vi "Initialize.vi"(8 "error in (no error)":errorcluster, 11 "UDP Thread UI in":refnum<class "UDP Thread User Interface.lvclass">) -> (0 "error out":errorcluster, 3 "UDP Thread UI out":refnum<class "UDP Thread User Interface.lvclass">)   [LabVIEW 2023, in "UDP.lvlib" / "UDP Thread User Interface.lvclass"]
uses:
  UDP Thread User Interface.lvclass
  C:/Users/Public/Documents/National Instruments/NI VeriStand 2023/Custom Devices/Data Sharing Framework/Linux_x64/DSF Core.lvlibp/Classes/User Interface/User Interface.lvclass
  Configuration/Thread/UDP Thread Configuration.lvclass
  C:/Users/Public/Documents/National Instruments/NI VeriStand 2023/Custom Devices/Data Sharing Framework/Linux_x64/DSF Core.lvlibp/Classes/Configuration/Configuration.lvclass
  Users/Public/Documents/National Instruments/NI VeriStand 2023/Custom Devices/Data Sharing Framework/Linux_x64/DSF Core.lvlibp/Classes/User Interface/User Interface.lvclass
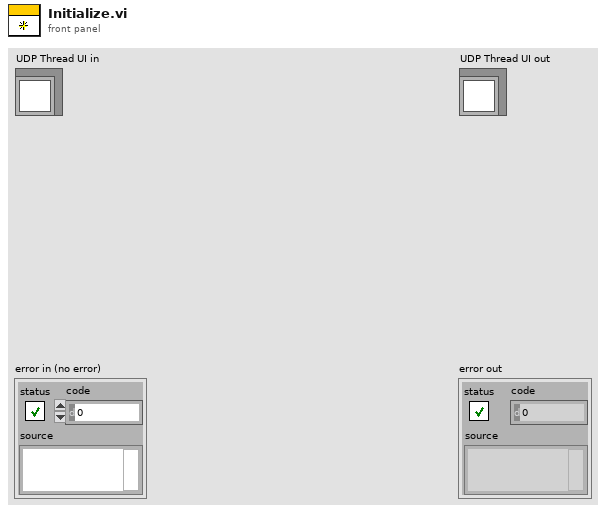
[diagram p1: front panel]
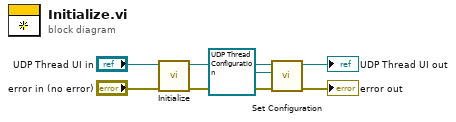
[diagram p0: block diagram]
diagram:
  n1 = call-parent "Initialize.vi"("error in (no error)"="error in (no error)", "User Interface in"="UDP Thread UI in") -> ("error out"=w4:errorcluster, "User Interface out"=w5:refnum<class "UDP Thread User Interface.lvclass">)  [unwired: 8 in]
  n2 = call "Set Configuration.vi"("error in (no error)"=w4, "configuration"=refnum<class "UDP Thread Configuration.lvclass"> refnum ("DSF Core.lvlib:DSF UDP Thread Configuration"), "User Interface in"=w5) -> ("error out"=→"error out":errorcluster, "User Interface out"=→"UDP Thread UI out":refnum<class "UDP Thread User Interface.lvclass">)  [unwired: 7 in]
